vi "Parse Sweep.vi"(0 "Path Group in":refnum<class "Path Group.lvclass">, 5 "Config Rows":string[][](array[string]), 11 "error in (no error)":errorcluster) -> (4 "Path Group out":refnum<class "Path Group.lvclass">, 15 "error out":errorcluster)   [LabVIEW 2023, in "RFCalAndFixtureCharact.Common.lvlib" / "Path Group.lvclass"]
uses:
  Path Group.lvclass
  RFCalAndFixtureCharact.Common.lvlib
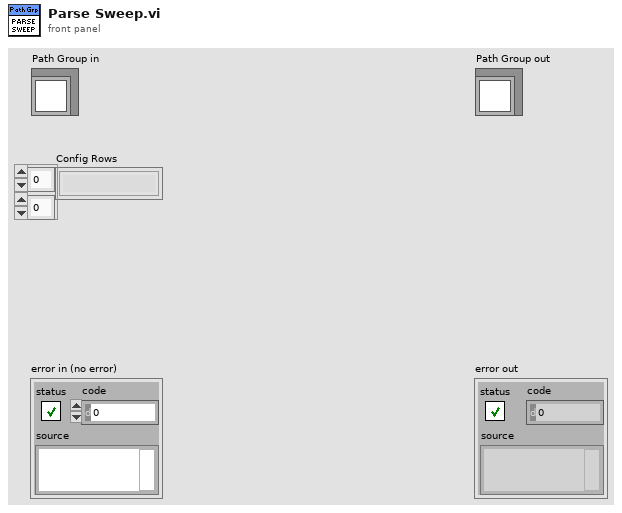
[diagram p1: front panel]
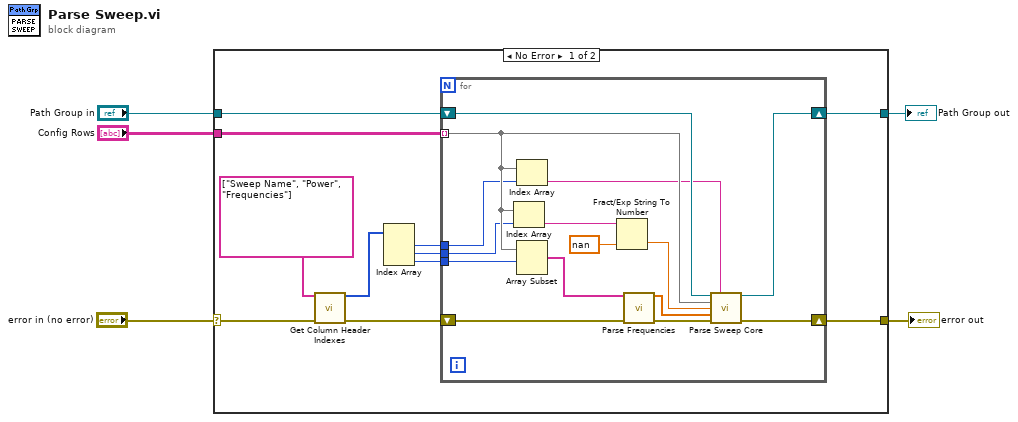
[diagram p0: block diagram]
diagram:
  n1 = case shown="No Error" "error in (no error)" {
    selector: "error in (no error)" -> [w10 w33]
    tunnel: [w13 w33] -> w4
    tunnel: [w15 w32] -> w2
    tunnel: "Path Group in" -> [w16 w32]
    tunnel: "Config Rows" -> [w14 _]
    frame No Error {
      n2 = call "Get Column Header Indexes.vi"("Column Header Names"=string[] ["Sweep Name", "Power", "Frequencies"], "error in"=w10) -> ("Column Header Indices"=w11:i32[], "error out"=w9:errorcluster)  [unwired: 11 in, 1 out]
      n3 = Index Array(array=w11) -> (element #1=w8:i32, element #2=w7:i32, element #3=w6:i32)  [unwired: 3 in]
      n4 = for {
        tunnel: w14 -> [w22] mode=indexing
        shift-right: [w30] -> w15
        shift-left: w16 -> [w31]
        shift-right: [w29] -> w13
        shift-left: w9 -> [w17]
        tunnel: w8 -> [w20]
        tunnel: w7 -> [w19]
        tunnel: w6 -> [w18]
        n5 = Index Array(array=w22, index=w19) -> (element=w26:string)
        n6 = Index Array(array=w22, index=w20) -> (element=w21:string)
        n7 = Array Subset(array=w22, index=w18) -> (w28:string[])  [unwired: 1 in]
        n8 = Fract/Exp String To Number(string=w26, default (0 dbl)=nan) -> (number=w25:dbl)  [unwired: 2 in, 1 out]
        n9 = call "Parse Frequencies.vi"("Frequencies in"=w28, "error in (no error)"=w17) -> ("Frequencies out"=w24:dbl[], "error out"=w27:errorcluster)  [unwired: 12 in]
        n10 = call-dynamic "Parse Sweep Core.vi"("Path Group in"=w31, "Sweep Name"=w21, "Config Rows"=w22, "Power"=w25, "Frequencies"=w24, "error in (no error)"=w27) -> ("Path Group out"=w30:refnum<class "Path Group.lvclass">, "error out"=w29:errorcluster)  [unwired: 8 in]
      }
    }
    frame Error {
    }
  }
  "error out" <- w4
  "Path Group out" <- w2
